vi "Update Configuration.vi"(8 "error in (no error)":errorcluster, 11 "CIFTemplatePlugin in":refnum<class "CIFTemplatePlugin.lvclass">) -> (0 "error out":errorcluster, 3 "CIFTemplatePlugin out":refnum<class "CIFTemplatePlugin.lvclass">)   [LabVIEW 2021, in "CIFTemplatePlugin.lvclass"]
uses:
  CIFTemplatePlugin.lvclass
  D:/dev/CIF-LVCore/src/CIFCore/Class/CIFCorePlugin.lvclass
  CIFCore/Class/CIFCorePlugin.lvclass/CIFCorePlugin.ctl
  CIFUtilities/CIFOutOfBand/CIFOutOfBand.lvclass/CIFOutOfBand.ctl
  CIFTemplatePlugin.lvclass/CIFTemplatePlugin.ctl
  CIFUtilities/CIFClocks/Core/Get Time.vi
  <vilib>/Utility/error.llb/Clear Errors.vi
  CIFCore/OOB/OOB_Rx/Receive/Read Configuration.vi
  CIFUtilities/CIFClocks/Time Conversion/LabVIEW Time to UTC Time.vi
  CIFCore/Common/Utilities/Add Error.vi
  CIFCore/OOB/OOB_Rx/Private/Read Payload.vi
  CIFCore/Common/Utilities/Append Error Location.vi
  CIFUtilities/CIFOutOfBand/Accessors/Read Local OOB Data.vi
  CIFCore/OOB/OOB_Rx/CIFCoreOOB_Rx.lvclass
  D:/dev/CIF-LVCore/src/CIFUtilities/CIFOutOfBand/CIFOutOfBand.lvclass
  CIFCore/Class/CIFCorePlugin.lvclass
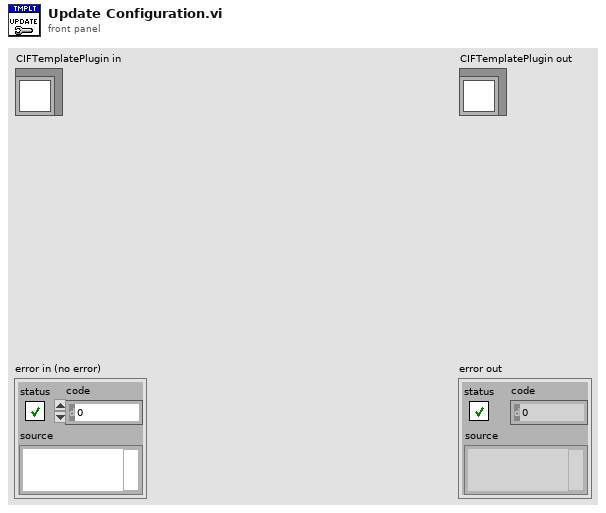
[diagram p1: front panel]
types:
  T1 = typedef "CIFTemplatePluginCommon.lvlib/Configuration.ctl" = cluster{"Common":T2, "Step":u64}
  T2 = typedef "CIFCoreCommon.lvlib/Common Plugin Configuration.ctl" = cluster{"Period (s)":dbl, "Offset (us)":i32, "ClockID":u8, "Priority":i32, "Processor":i32}
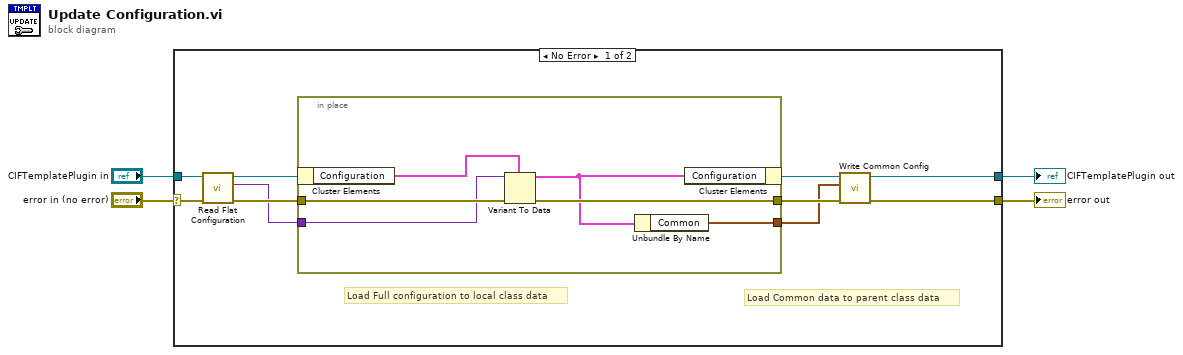
[diagram p0: block diagram]
diagram:
  n1 = case shown="No Error" "error in (no error)" {
    selector: "error in (no error)" -> [w12 w21]
    tunnel: "CIFTemplatePlugin in" -> [w13 w22]
    tunnel: [w5 w22] -> w1
    tunnel: [w6 w21] -> w3
    frame No Error {
      # "Load Common data to parent class data"
      # "Load Full configuration to local class data"
      n2 = call "Read Flat Configuration.vi"("error in (no error)"=w12, "CIFTemplateNode in"=w13) -> ("error out"=w11:errorcluster, "Configuration"=w10:variant, "CIFTemplateNode out"=w9:refnum<class "CIFTemplatePlugin.lvclass">)  [unwired: 7 in]
      n3 = in-place {
        in-place-border: [w20] -> w14
        in-place-border: w11 -> [w19]
        in-place-border: w10 -> [w18]
        in-place-border: [w16] -> w8
        n4 = in-place-cluster #1(w9) -> ("Configuration"=w17:T1)
        n5 = Variant To Data(error in=w19, type=w17, Variant=w18) -> (data=w15:T1, error out=w20:errorcluster)
        n6 = Unbundle By Name(w15) -> ("Common"=w16:T2)
        n7 = in-place-cluster #1("Configuration"=w15) -> (w7:refnum<class "CIFTemplatePlugin.lvclass">)
      }
      n8 = call "Write Common Config.vi"("error in (no error)"=w14, "Common"=w8, "CIFTemplateNode in"=w7) -> ("error out"=w6:errorcluster, "CIFTemplateNode out"=w5:refnum<class "CIFTemplatePlugin.lvclass">)  [unwired: 7 in]
    }
    frame Error {
    }
  }
  "error out" <- w3
  "CIFTemplatePlugin out" <- w1
